vi "rad_Save Config.vi"(8 "error in (no error":errorcluster, 11 "State":T1 {"Targets Information"."Primary NIC"."IP Address Request Mode" items=["Static"=1, "DHCP/Link-Local"=2, "Link-Local Only"=4, "DHCP Only"=8]}) -> (0 "error out":errorcluster, 2 "Configuration File Path":path)   [LabVIEW 2016]
uses:
  TypeDefs/rad_State Data.ctl
  Targets/TypeDefs/rad_Targets Settings.ctl
  Targets/TypeDefs/rad_Target Information.ctl
  Targets/TypeDefs/rad_Target Network Settings.ctl
  App Images/TypeDefs/rad_App Images Settings.ctl
  App Images/TypeDefs/rad_AppImage Information.ctl
  App Images/TypeDefs/rad_Application Image Properties.ctl
  App Images/TypeDefs/rad_FPGA Properties.ctl
  App Images/TypeDefs/rad_FPGA Flash Properties.ctl
  <vilib>/Utility/config.llb/Write Key (Path).vi
  rad_Globals.vi
  <vilib>/Utility/config.llb/Write Key (String).vi
  <vilib>/Utility/config.llb/Write Key (Boolean).vi
  <vilib>/Utility/config.llb/Write Key (I32).vi
  <vilib>/Utility/config.llb/NI_LVConfig.lvlib
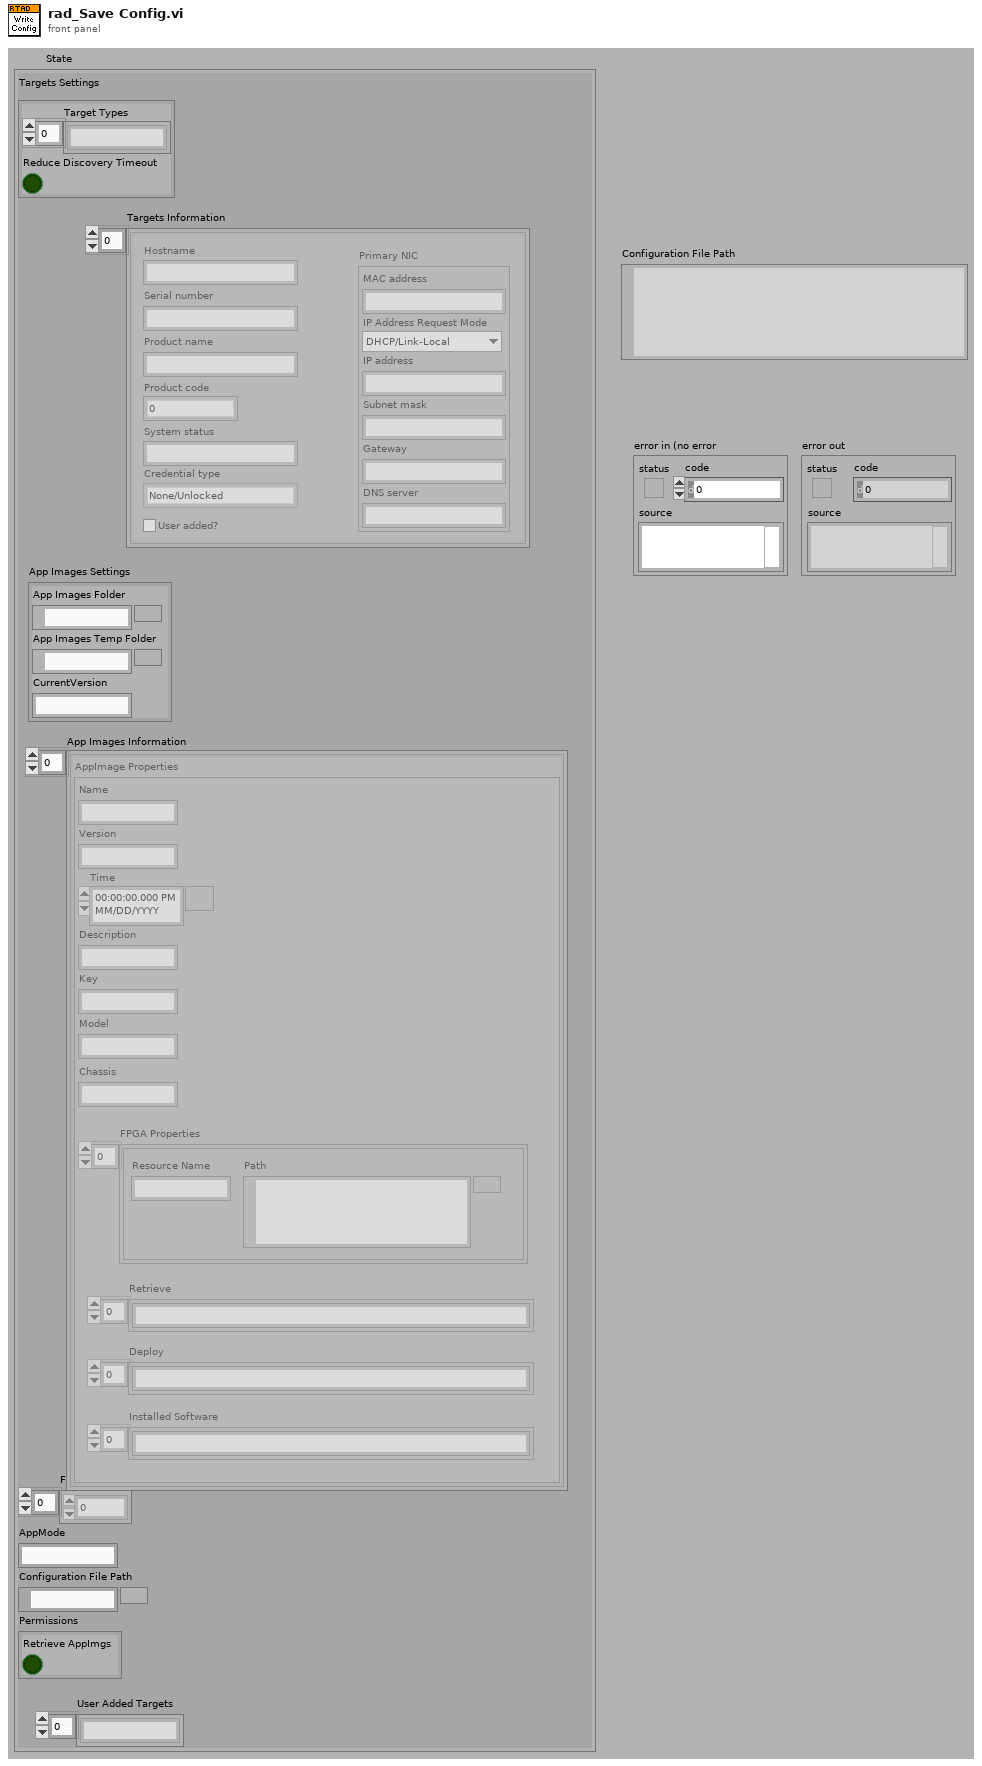
[diagram p1: front panel]
types:
  T1 = typedef "rad_State Data.ctl" = cluster{"Targets Settings":T2, "Targets Information":T3[], "App Images Settings":T5, "App Images Information":T6[], "Filtered Targets":i32[], "AppMode":string, "Configuration File Path":path, "Permissions":cluster{"Retrieve AppImgs":bool}, "User Added Targets":string[]}
  T2 = typedef "rad_Targets Settings.ctl" = cluster{"Target Types":string[], "Reduce Discovery Timeout":bool}
  T3 = typedef "rad_Target Information.ctl" = cluster{"Hostname":string, "Serial number":string, "Product name":string, "Product code":i32, "System status":string, "Credential type":enum16{"None/Unlocked", "FTP Password", "NIAuth Credentials"}, "User added?":bool, "Primary NIC":T4}
  T4 = typedef "rad_Target Network Settings.ctl" = cluster{"MAC address":string, "IP Address Request Mode":i32, "IP address":string, "Subnet mask":string, "Gateway":string, "DNS server":string}
  T5 = typedef "rad_App Images Settings.ctl" = cluster{"App Images Folder":path, "App Images Temp Folder":path, "CurrentVersion":string}
  T6 = typedef "rad_AppImage Information.ctl" = cluster{"AppImage Properties":T7, "AppImage Path":path}
  T7 = typedef "rad_Application Image Properties.ctl" = cluster{"Name":string, "Version":string, "Time":timestamp, "Description":string, "Key":string, "Chassis":string, "FPGA Properties":T8, "Model":string, "Retrieve":string[], "Deploy":string[], "Installed Software":string[]}
  T8 = typedef "rad_FPGA Properties.ctl" = T9[]
  T9 = typedef "rad_FPGA Flash Properties.ctl" = cluster{"Resource Name":string, "Path":path}
  T10 = typedef "NI_LVConfig.lvlib/Config Data RefNum.ctl" = refnum<k1>
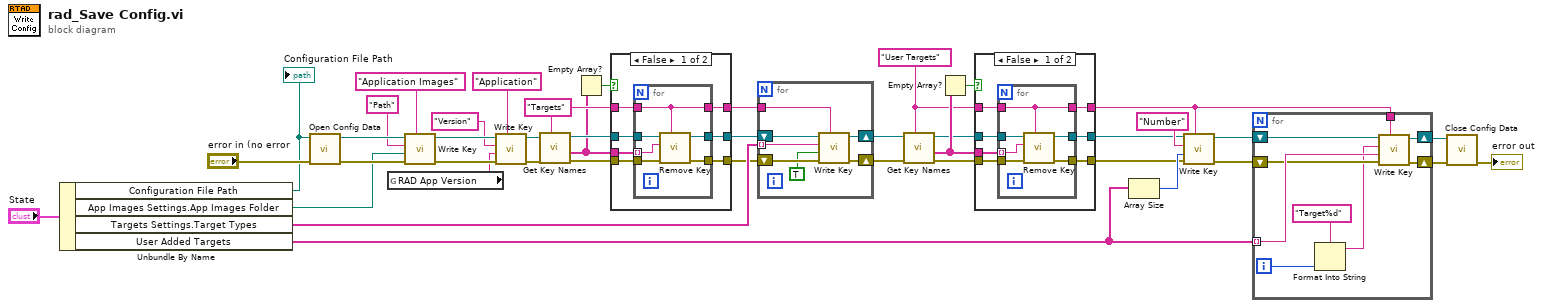
[diagram p0: block diagram]
diagram:
  w11 = "User Targets" ("section")
  w36 = "Targets" ("section")
  n1 = Unbundle By Name("State") -> ("Configuration File Path"=w1:path, "App Images Settings.App Images Folder"=w38:path, "Targets Settings.Target Types"=w35:string[], "User Added Targets"=w10:string[])
  "Configuration File Path" <- w1
  n2 = call <vilib>:"Open Config Data.vi"("error in (no error)"="error in (no error", "configuration file path"=w1) -> ("error out"=w41:errorcluster, "refnum"=w40:T10)  [unwired: 7 in, 1 out]
  n3 = global read "rad_Globals.vi" "RAD App Version"() -> (w3:string)
  n4 = call-poly <vilib>:"Write Key.vi"("section"="Application Images", "error in (no error)"=w41, "value"=w38, "key"="Path", "refnum"=w40) -> ("error out"=w8:errorcluster, "refnum out"=w9:T10)  [unwired: 1 in, 4 out]
  n5 = call-poly <vilib>:"Write Key.vi"("section"="Application", "error in (no error)"=w8, "value"=w3, "key"="Version", "refnum"=w9) -> ("error out"=w4:errorcluster, "refnum out"=w5:T10)  [unwired: 1 in, 4 out]
  n6 = call <vilib>:"Get Key Names.vi"("section"=w36, "error in (no error)"=w4, "refnum"=w5) -> ("error out"=w37:errorcluster, "key names"=w31:string[], "refnum out"=w32:T10)  [unwired: 6 out]
  n7 = Empty Array?(array=w31) -> (empty?=w30:bool)
  n8 = case shown="False" w30 {
    tunnel: w37 -> [w49 w56]
    tunnel: w31 -> [w48 _]
    tunnel: w36 -> [w47 w58]
    tunnel: w32 -> [w46 w57]
    tunnel: [w43 w58] -> w29
    tunnel: [w45 w57] -> w28
    tunnel: [w44 w56] -> w27
    frame False {
      n9 = for {
        tunnel: w49 -> [w55]
        tunnel: w46 -> [w52]
        tunnel: w48 -> [w53] mode=indexing
        tunnel: w47 -> [w54]
        tunnel: [w54] -> w43
        tunnel: [w51] -> w44
        tunnel: [w50] -> w45
        n10 = call <vilib>:"Remove Key.vi"("section"=w54, "error in (no error)"=w55, "key"=w53, "refnum"=w52) -> ("error out"=w51:errorcluster, "refnum out"=w50:T10)  [unwired: 6 out]
      }
    }
    frame True {
    }
  }
  n11 = for {
    tunnel: w35 -> [w62] mode=indexing
    tunnel: w29 -> [w59]
    shift-right: [w61] -> w16
    shift-left: w28 -> [w65]
    shift-right: [w60] -> w15
    shift-left: w27 -> [w64]
    n12 = call-poly <vilib>:"Write Key.vi"("section"=w59, "error in (no error)"=w64, "value"=TRUE, "key"=w62, "refnum"=w65) -> ("error out"=w60:errorcluster, "refnum out"=w61:T10)  [unwired: 1 in, 4 out]
  }
  n13 = call <vilib>:"Get Key Names.vi"("section"=w11, "error in (no error)"=w15, "refnum"=w16) -> ("error out"=w17:errorcluster, "key names"=w19:string[], "refnum out"=w18:T10)  [unwired: 6 out]
  n14 = Empty Array?(array=w19) -> (empty?=w20:bool)
  n15 = case shown="False" w20 {
    tunnel: w17 -> [w72 w79]
    tunnel: w19 -> [w71 _]
    tunnel: w11 -> [w70 w81]
    tunnel: w18 -> [w69 w80]
    tunnel: [w66 w81] -> w14
    tunnel: [w68 w80] -> w13
    tunnel: [w67 w79] -> w12
    frame False {
      n16 = for {
        tunnel: w72 -> [w78]
        tunnel: w69 -> [w75]
        tunnel: w71 -> [w76] mode=indexing
        tunnel: w70 -> [w77]
        tunnel: [w77] -> w66
        tunnel: [w74] -> w67
        tunnel: [w73] -> w68
        n17 = call <vilib>:"Remove Key.vi"("section"=w77, "error in (no error)"=w78, "key"=w76, "refnum"=w75) -> ("error out"=w74:errorcluster, "refnum out"=w73:T10)  [unwired: 6 out]
      }
    }
    frame True {
    }
  }
  n18 = Array Size(array=w10) -> (size(s)=w26:i32)
  n19 = call-poly <vilib>:"Write Key.vi"("section"=w14, "error in (no error)"=w12, "value"=w26, "key"="Number", "refnum"=w13) -> ("error out"=w23:errorcluster, "refnum out"=w24:T10)  [unwired: 1 in, 4 out]
  n20 = for {
    tunnel: w10 -> [w88] mode=indexing
    tunnel: w14 -> [w89]
    shift-right: [w86] -> w22
    shift-left: w23 -> [w87]
    shift-right: [w85] -> w21
    shift-left: w24 -> [w90]
    i -> [w83]
    n21 = Format Into String(format string="Target%d", w83) -> (resulting string=w82:string)  [unwired: 2 in, 1 out]
    n22 = call-poly <vilib>:"Write Key.vi"("section"=w89, "error in (no error)"=w87, "value"=w88, "key"=w82, "refnum"=w90) -> ("error out"=w86:errorcluster, "refnum out"=w85:T10)  [unwired: 1 in, 4 out]
  }
  n23 = call <vilib>:"Close Config Data.vi"("error in (no error)"=w22, "refnum"=w21) -> ("error out"=→"error out":errorcluster)  [unwired: 1 in, 8 out]
